vi "__read_temp_1ch.vi"(2 "ch":i32, 3 "GIPBÔ":string="18") -> (1 "input A":dbl format="%.4f")   [LabVIEW 2017]
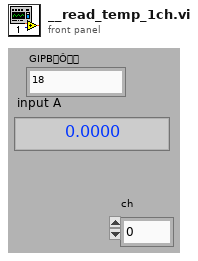
[diagram p1: front panel]
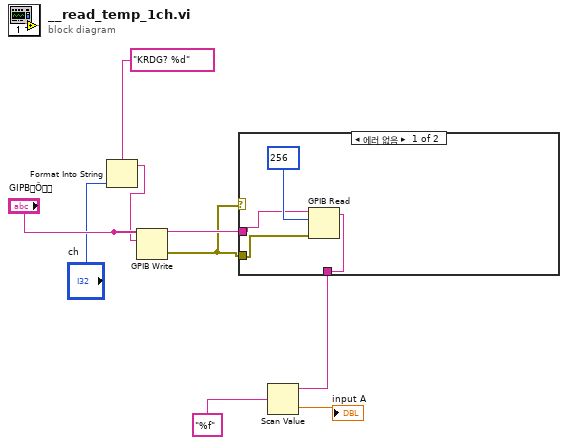
[diagram p0: block diagram]
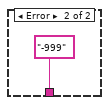
[diagram p2: hidden frame]
diagram:
  n1 = Format Into String(format string="KRDG? %d", "ch") -> (resulting string=w1:string)  [unwired: 2 in, 1 out]
  n2 = GPIB Write(0:"GIPBÔ", 1:w1) -> (6:w4:errorcluster)  [unwired: 3 in, 1 out]
  n3 = case shown="에러 없음" w4 {
    tunnel: w4 -> [w10 _]
    tunnel: "GIPBÔ" -> [w11 _]
    tunnel: [w9 "-999"] -> w5
    frame No Error {
      n4 = GPIB Read(0:w11, 1:256, 3:w10) -> (5:w9:string)  [unwired: 2 in, 2 out]
    }
    frame Error {
    }
  }
  n5 = Scan Value(string=w5, format string="%f" ("Œ`Ž®•¶Žš—ñ")) -> (value=→"input A":dbl)  [unwired: 1 in, 1 out]
